vi "Convertpourcentmode2.vi"() -> ()   [LabVIEW 2015]
panel:
  in  "input variable":i16
  out "output variable":i16
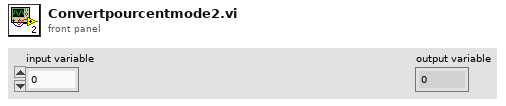
[diagram p1: front panel]
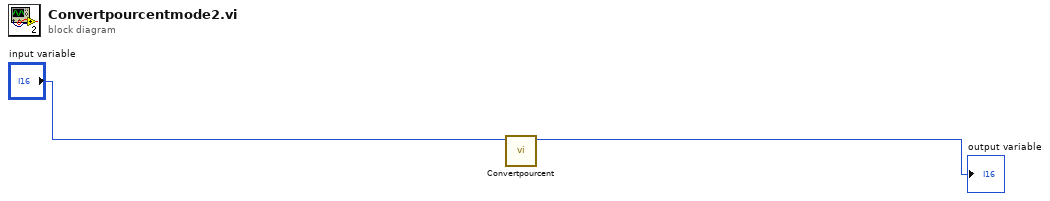
[diagram p0: block diagram]
diagram:
  n1 = call "Convertpourcent.vi"("input variable"="input variable") -> ("output variable"=→"output variable":i16)  [unwired: 10 in]
